vi "Shut Down Device.vi"(8 "error in (no error)":errorcluster, 11 "TE2000 in":refnum<class "Eclipse TI.lvclass">) -> (0 "error out":errorcluster, 3 "TE2000 out":refnum<class "Eclipse TI.lvclass">)   [LabVIEW 2015, in "Eclipse TI.lvlib" / "Eclipse TI.lvclass"]
uses:
  Eclipse TI.lvclass
  Eclipse TI.lvclass/Eclipse TI.ctl
  Device/Device.lvclass
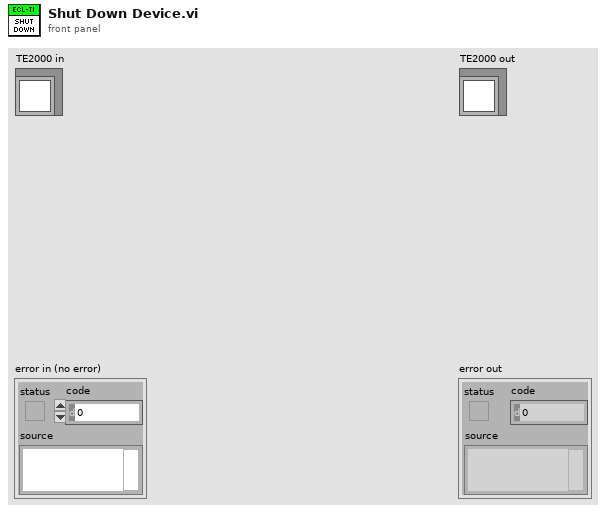
[diagram p1: front panel]
types:
  T1 = typedef "Microscope Type.ctl" = enum16{"TE2000", "Eclipse Ti"}
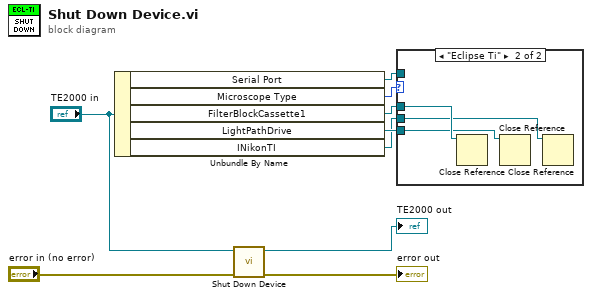
[diagram p0: block diagram]
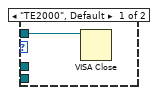
[diagram p2: hidden frame]
diagram:
  n1 = Unbundle By Name("TE2000 in") -> ("Serial Port"=w5:refnum<visa-resource-name>, "Microscope Type"=w4:T1, "FilterBlockCassette1"=w3:refnum<k7>, "LightPathDrive"=w2:refnum<k7>, "INikonTI"=w1:refnum<k7>)
  n2 = call-parent "Shut Down Device.vi"("error in (no error)"="error in (no error)", "Device in"="TE2000 in") -> ("error out"=→"error out":errorcluster, "Device out"=→"TE2000 out":refnum<class "Eclipse TI.lvclass">)  [unwired: 8 in]
  n3 = case shown="\"Eclipse Ti\"" w4 {
    tunnel: w5 -> [w10 _]
    tunnel: w3 -> [_ w13]
    tunnel: w2 -> [_ w12]
    tunnel: w1 -> [_ w11]
    frame "TE2000", Default {
      n4 = VISA Close(VISA resource name=w10) -> ()  [unwired: 1 in, 1 out]
    }
    frame "Eclipse Ti" {
      n5 = Close Reference(reference=w13) -> ()  [unwired: 1 in, 1 out]
      n6 = Close Reference(reference=w12) -> ()  [unwired: 1 in, 1 out]
      n7 = Close Reference(reference=w11) -> ()  [unwired: 1 in, 1 out]
    }
  }
